vi "USBTC08GetInfo.vi"(8 "error in (no error)":errorcluster, 11 "Handle in":i16) -> (0 "error out":errorcluster, 1 "Unit Info":T1, 3 "Handle out":i16)   [LabVIEW 2009]
uses:
  usbtc08.dll
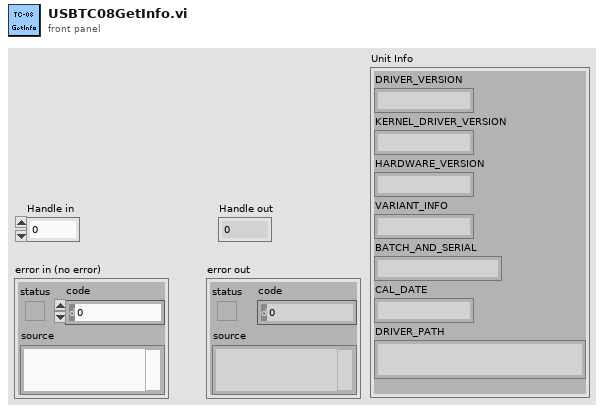
[diagram p1: front panel]
types:
  T1 = cluster{"DRIVER_VERSION":string, "KERNEL_DRIVER_VERSION":string, "HARDWARE_VERSION":string, "VARIANT_INFO":string, "BATCH_AND_SERIAL":string, "CAL_DATE":string, "DRIVER_PATH":string, "[7]":string, "[8]":string, "[9]":string, "[10]":string, "[11]":string, "[12]":string, "[13]":string, "[14]":string}
  T2 = cluster{"[0]":string, "[1]":string, "[2]":string, "[3]":string, "[4]":string, "[5]":string, "[6]":string, "[7]":string, "[8]":string, "[9]":string, "[10]":string, "[11]":string, "[12]":string, "[13]":string, "[14]":string}
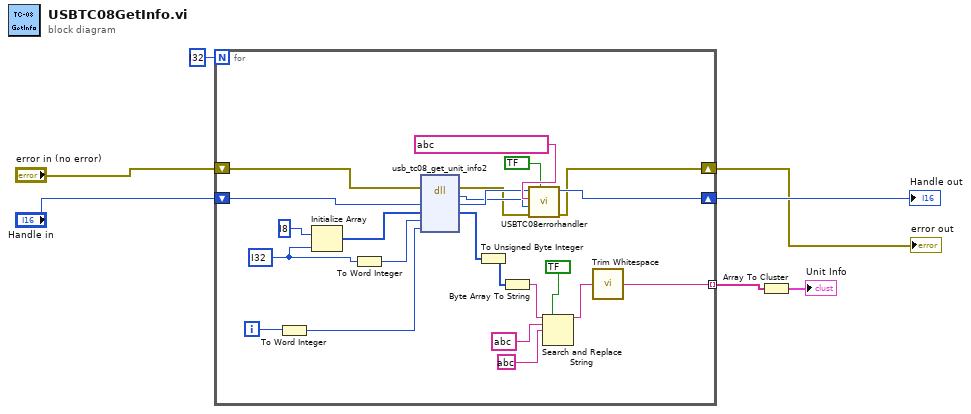
[diagram p0: block diagram]
diagram:
  n1 = for {
    N: i32 ? -> [_]
    shift-right: [w30] -> w7
    shift-left: "Handle in" -> [w28]
    shift-right: [w29] -> w6
    shift-left: "error in (no error)" -> [w24]
    tunnel: [w11] -> w2 mode=indexing
    i -> [w18]
    w19 = i32 ? ("dimension size")
    n2 = To Word Integer(number=w18) -> (16bit integer=w17:i16)
    n3 = Initialize Array(i8 ? ("element"), w19) -> (w22:i8[])
    n4 = To Word Integer(number=w19) -> (16bit integer=w20:i16)
    n5 = dll-call lib="usbtc08.dll" fn="usb_tc08_get_unit_info2" ("Set Mains")(error in=w24, "Handle"=w28, "string"=w22, "string_length"=w20, "line"=w17) -> (error out=w23:errorcluster, "Return"=w25:i16, "Handle"=w26:i16, "string"=w13:i8[])  [unwired: 4 in, 1 out]
    n6 = To Unsigned Byte Integer(number=w13) -> (unsigned 8bit integer=w12:u8[])
    n7 = Byte Array To String(unsigned byte array=w12) -> (string=w9:string)
    n8 = call "USBTC08errorhandler.vi"("Close unit"=bool ?, "error in (no error)"=w23, "Return"=w25, "API function"=string ?, "Handle in"=w26) -> ("error out"=w29:errorcluster, "Handle out"=w30:i16)  [unwired: 5 in]
    n9 = Search and Replace String(replace all?=bool ? ("replace all? (F)"), input string=w9, search string=string ?, replace string=string ?) -> (result string=w10:string)  [unwired: 4 in, 3 out]
    n10 = call <vilib>:"Trim Whitespace.vi"("string"=w10) -> ("trimmed string"=w11:string)  [unwired: 1 in]
  }
  "Handle out" <- w7
  "error out" <- w6
  n11 = Array To Cluster(array=w2) -> (cluster=→"Unit Info":T2)
